vi "Deinit.vi"(8 "error in (no error)":errorcluster, 11 "UI in":refnum<class "UI.lvclass">) -> (0 "error out":errorcluster)   [LabVIEW 2020, in "AR Example.lvlib" / "UI.lvclass"]
uses:
  UI.lvclass
  UI.lvclass/UI.ctl
  Calibration Board Events.ctl
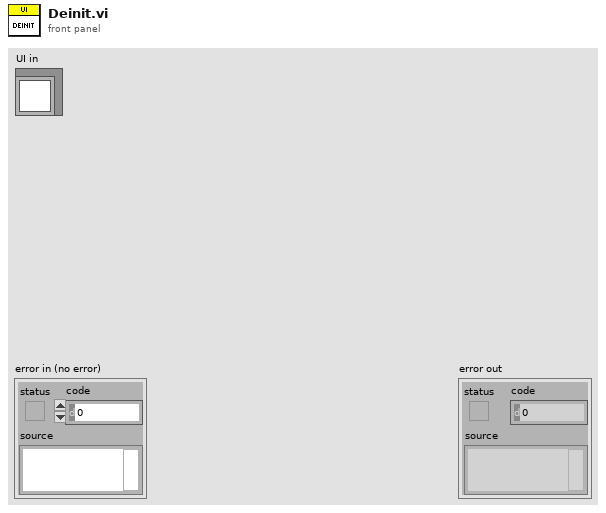
[diagram p1: front panel]
types:
  T1 = typedef "AR Example.lvlib/UI.lvclass/Calibration Board Events.ctl" = enum16{"Show Panel", "Hide Panel", "Exit"}
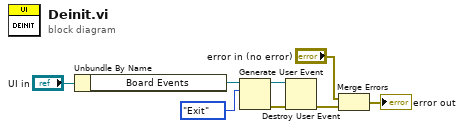
[diagram p0: block diagram]
diagram:
  n1 = Unbundle By Name("UI in") -> ("Board Events"=w6:refnum<user-event>)
  n2 = Generate User Event(user event=w6, event data cluster=Calibration_Board_Events."Exit" ("event data")) -> (user event out=w2:refnum<user-event>, error out=w3:errorcluster)  [unwired: 2 in]
  n3 = Destroy User Event(user event=w2, error in=w3) -> (error out=w1:errorcluster)
  n4 = Merge Errors("error in (no error)", w1) -> (→"error out":errorcluster)
